vi "CheckSum (SubVI).vi"(10 "String":string="Comms to SEND", 11 "Simulate error":bool) -> (2 "Numeric":u8, 3 "string":string)   [LabVIEW 2013]
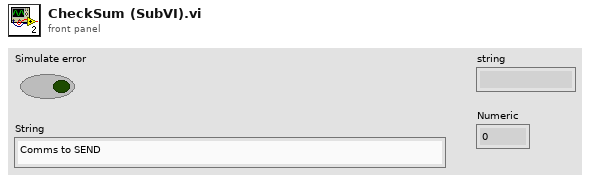
[diagram p1: front panel]
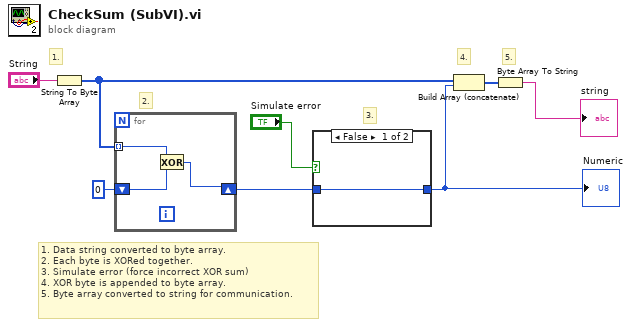
[diagram p0: block diagram]
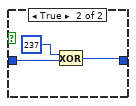
[diagram p2: hidden frame]
diagram:
  # "3."
  # "5."
  # "4."
  # "2."
  # "1."
  # "1. Data string converted to byte array.\n2. Each byte is XORed together.\n3. Simulate error (force incorrect XOR sum)\n4. XOR byte is appended to byte array.\n5. Byte array converted to string for communication."
  n1 = String To Byte Array(string="String") -> (unsigned byte array=w2:u8[])
  n2 = for {
    tunnel: w2 -> [w11] mode=indexing
    shift-right: [w9] -> w7
    shift-left: u8 0 -> [w10]
    n3 = Exclusive Or(1:w10, 2:w11) -> (0:w9:u8)
  }
  n4 = case shown="False" "Simulate error" {
    tunnel: [w12 w14] -> w6
    tunnel: w7 -> [w12 w15]
    frame False {
    }
    frame True {
      n5 = Exclusive Or(1:w15, 2:u8 237 ("x")) -> (0:w14:u8)
    }
  }
  "Numeric" <- w6
  n6 = Build Array (concatenate)(w2, w6) -> (w1:u8[])
  n7 = Byte Array To String(unsigned byte array=w1) -> (string=→"string":string)
